vi "mDrive Send Command.vi"(6 "error in (no error)":errorcluster, 7 "Extra":string, 8 "Command":T1(ring), 9 "VISA resource name":refnum<visa-resource-name>="COM1") -> (0 "error out":errorcluster, 2 "read buffer":string, 3 "VISA resource name out":refnum<visa-resource-name>)   [LabVIEW 2009]
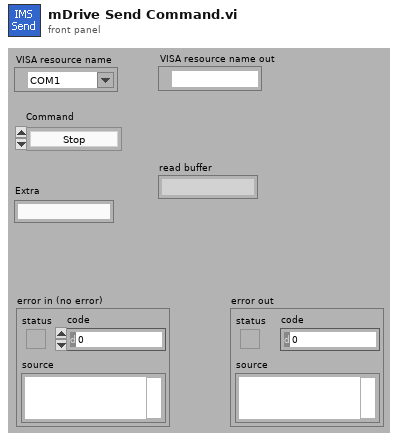
[diagram p1: front panel]
types:
  T1 = enum16{"Stop", "Reset", "Run Current", "Holding Current", "Accel Rate", "Decel Rate", "Move to Relative Position", "Move to Absolute Position", "Echo Mode", "Print Parameter", "Send String", "Microstep Resolution", "Set Current Position", "Max Velocity"}
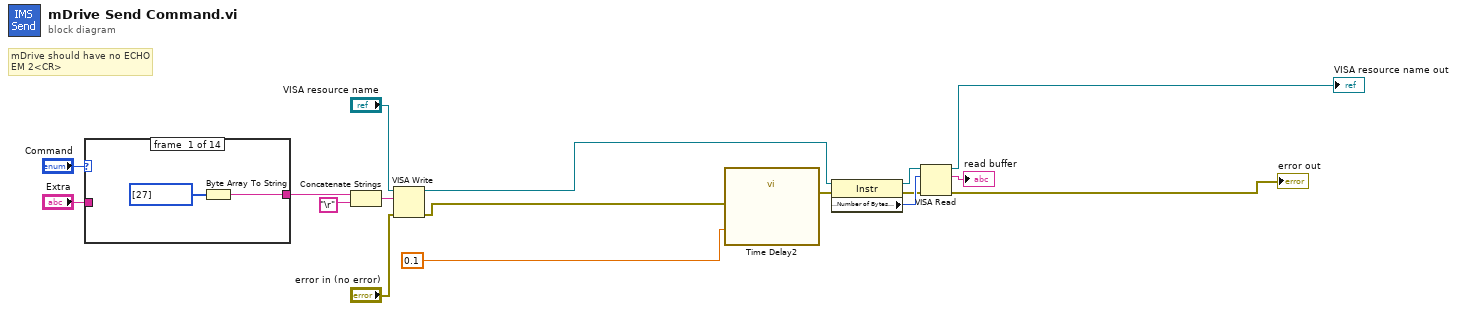
[diagram p0: block diagram]
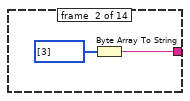
[diagram p2: hidden frame]
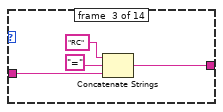
[diagram p3: hidden frame]
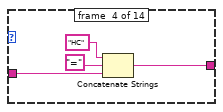
[diagram p4: hidden frame]
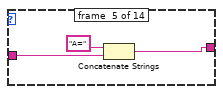
[diagram p5: hidden frame]
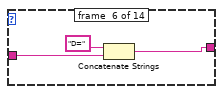
[diagram p6: hidden frame]
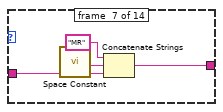
[diagram p7: hidden frame]
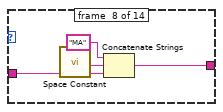
[diagram p8: hidden frame]
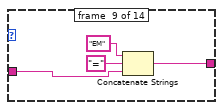
[diagram p9: hidden frame]
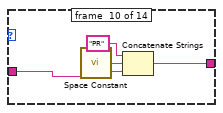
[diagram p10: hidden frame]
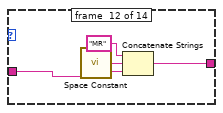
[diagram p12: hidden frame]
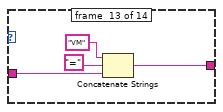
[diagram p13: hidden frame]
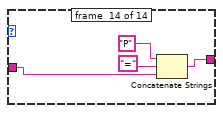
[diagram p14: hidden frame]
diagram:
  # "mDrive should have no ECHO\nEM 2<CR>"
  n1 = case shown="\"Move to Relative Position\"" "Command" {
    tunnel: "Extra" -> [_ _ w23 w27 w30 w34 w37 w41 w44 w48 w52 w53 w58 w62]
    tunnel: [w18 w21 w24 w28 w31 w33 w36 w40 w45 w49 w52 w54 w57 w61] -> w10
    frame #0 {
      n2 = Byte Array To String(unsigned byte array=u8[] [27]) -> (string=w18:string)
    }
    frame #1 {
      n3 = Byte Array To String(unsigned byte array=u8[] [3]) -> (string=w21:string)
    }
    frame #2 {
      n4 = Concatenate Strings("RC", "=", w23) -> (w24:string)
    }
    frame #3 {
      n5 = Concatenate Strings("HC", "=", w27) -> (w28:string)
    }
    frame #4 {
      n6 = Concatenate Strings("A=", w30) -> (w31:string)
    }
    frame #5 {
      n7 = Concatenate Strings("D=", w34) -> (w33:string)
    }
    frame #6 {
      n8 = call <vilib>:"Space Constant.vi"() -> ("String"=w38:string)
      n9 = Concatenate Strings("MR", w38, w37) -> (w36:string)
    }
    frame #7 {
      n10 = call <vilib>:"Space Constant.vi"() -> ("String"=w42:string)
      n11 = Concatenate Strings("MA", w42, w41) -> (w40:string)
    }
    frame #8 {
      n12 = Concatenate Strings("EM", "=", w44) -> (w45:string)
    }
    frame #9 {
      n13 = call <vilib>:"Space Constant.vi"() -> ("String"=w50:string)
      n14 = Concatenate Strings("PR", w50, w48) -> (w49:string)
    }
    frame #10 {
    }
    frame #11 {
      n15 = call <vilib>:"Space Constant.vi"() -> ("String"=w55:string)
      n16 = Concatenate Strings("MR", w55, w53) -> (w54:string)
    }
    frame #12 {
      n17 = Concatenate Strings("VM", "=", w58) -> (w57:string)
    }
    frame #13 {
      n18 = Concatenate Strings("P", "=", w62) -> (w61:string)
    }
  }
  n19 = Concatenate Strings(w10, "\r") -> (w15:string)
  n20 = VISA Write(VISA resource name="VISA resource name", write buffer=w15, error in (no error)="error in (no error)") -> (VISA resource name out=w4:refnum<visa-resource-name>, error out=w3:errorcluster)  [unwired: 1 out]
  n21 = call "Time Delay2"("error in (no error)"=w3, "Delay Time (s)"=0.1) -> ("error out"=w6:errorcluster)  [unwired: 9 in]
  n22 = property class="Instr"(reference=w4, error in=w6) -> (reference out=w8:refnum<visa-resource-name>, error out=w7:errorcluster, "Serial Settings:Number of Bytes at Serial Port"=w9:u32)
  n23 = VISA Read(VISA resource name=w8, byte count=w9, error in (no error)=w7) -> (VISA resource name out=→"VISA resource name out":refnum<visa-resource-name>, read buffer=→"read buffer":string, error out=→"error out":errorcluster)  [unwired: 1 out]
